vi "AF_4.0.0_Actor Core2.vi"(8 "error in":errorcluster, 11 "Actor in":refnum<class "Actor1_GUI_N_4.0.0.lvclass">) -> (0 "error out":errorcluster, 3 "Actor out(KEEP)":refnum<class "Actor.lvclass">)   [LabVIEW 2020]
doc: "This is Actor Core.vi, the main message handling loop for Actors. An actor usually just sits in this loop and processes messages as they arrive. Any error returned by the message Do.vi call will stop the loop, with error code 43 as the cannonical signal to stop with no error sent to caller. Descendants may override that in Handle Error.vi."
uses:
  <vilib>/ActorFramework/Actor/Actor.lvclass
  <vilib>/ActorFramework/Stop Msg/Stop Msg.lvclass
  Actor1_GUI_N_4.0.0/Actor1_GUI_N_4.0.0_class/Actor1_GUI_N_4.0.0.lvclass
panel:
  out "StopLoop(Hidden)":bool
  in  "Stop":bool
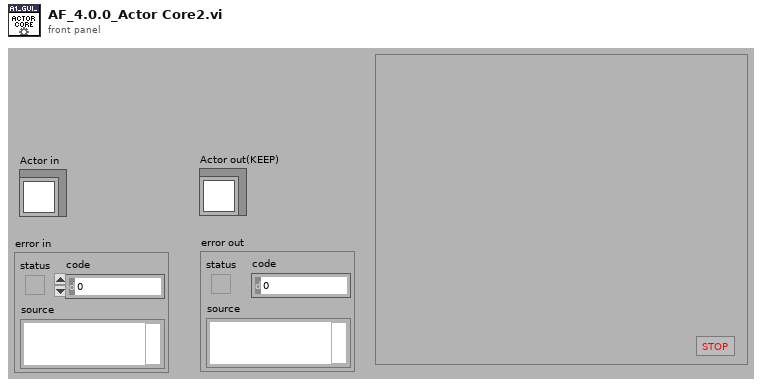
[diagram p1: front panel]
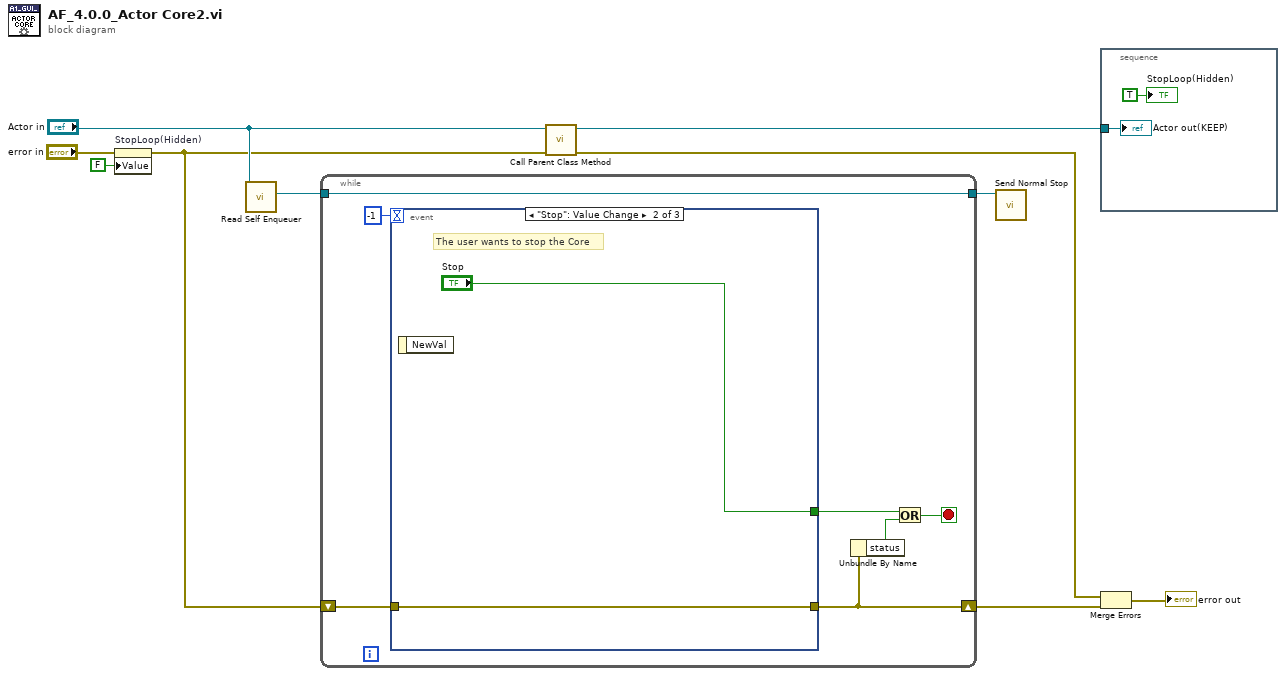
[diagram p0: block diagram]
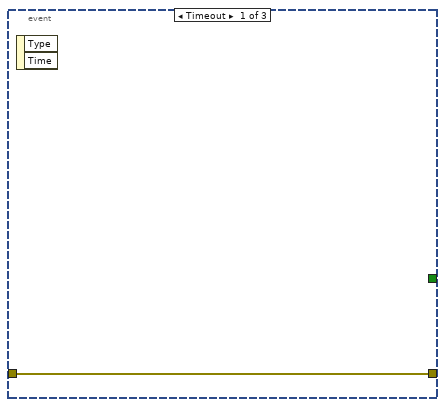
[diagram p2: hidden frame]
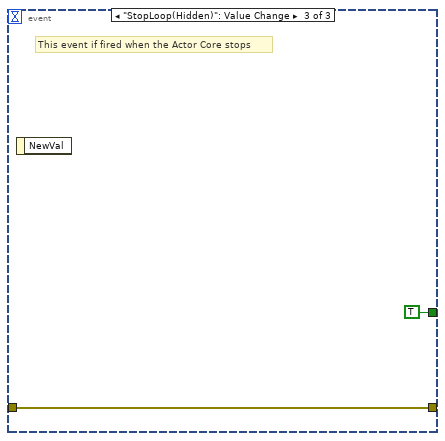
[diagram p3: hidden frame]
diagram:
  n1 = property on="StopLoop(Hidden)" class="Bool (strict)"(error in="error in", "Value"=FALSE ("Stop")) -> (error out=w5:errorcluster)  [unwired: 1 in, 1 out]
  n2 = call <vilib>:"Read Self Enqueuer.vi"("Actor"="Actor in") -> ("Self Enqueuer"=w2:refnum<class "Message Enqueuer.lvclass">)  [unwired: 10 in]
  n3 = while {
    tunnel: w2 -> [w11]
    shift-right: [w12] -> w10
    shift-left: w5 -> [w17]
    tunnel: [w11] -> w1
    stop <- w13 stop-if-true
    n4 = event shown="[1] \"Stop\": Value Change" {
      selector: _ -> [_ _ _]
      dyn-events: _ -> [_ _ _]
      timeout: -1 -> [_ _ _]
      tunnel: w17 -> [w18 w20 w22]
      tunnel: [w18 w20 w22] -> w12
      tunnel: [_ "Stop" TRUE ("Stop")] -> w14
      event Timeout {
        n5 = event-data() -> ()  [unwired: 1 in, 2 out]
      }
      event "Stop": Value Change {
        # "The user wants to stop the Core"
        n6 = event-data() -> ()  [unwired: 1 in, 1 out]
      }
      event "StopLoop(Hidden)": Value Change {
        # "This event if fired when the Actor Core stops"
        n7 = event-data() -> ()  [unwired: 1 in, 1 out]
      }
    }
    n8 = Unbundle By Name(w12) -> ("status"=w15:bool)
    n9 = Or(x=w14, y=w15) -> (x .or. y?=w13:bool)
  }
  n10 = call-parent "Call Parent Class Method"("error in"=w5, "Actor"="Actor in") -> ("error out"=w9:errorcluster, "Actor out"=w3:refnum<class "Actor.lvclass">)  [unwired: 8 in]
  n11 = call <vilib>:"Send Normal Stop.vi"("Message Enqueuer"=w1) -> ()  [unwired: 10 in, 1 out]
  n12 = stacked-sequence {
    tunnel: w3 -> [w24]
    frame #0 {
      "Actor out(KEEP)" <- w24
      "StopLoop(Hidden)" <- TRUE ("StopLoop(Hidden)")
    }
  }
  n13 = Merge Errors(w9, w10) -> (→"error out":errorcluster)
